vi "FSK_Sampling.vi"(8 "error in (no error)":errorcluster caption="错误输入（无错误）", 9 "pos":dbl format="%#_13g", 10 "RecvFskDemod":dbl[](array[numeric]) format="%#_13g", 11 "PathIn":path) -> (0 "error out":errorcluster caption="错误输出", 2 "RecvSymbolSampled":dbl[](array[numeric]) format="%#_13g", 3 "PathOut":path)   [LabVIEW 2015]
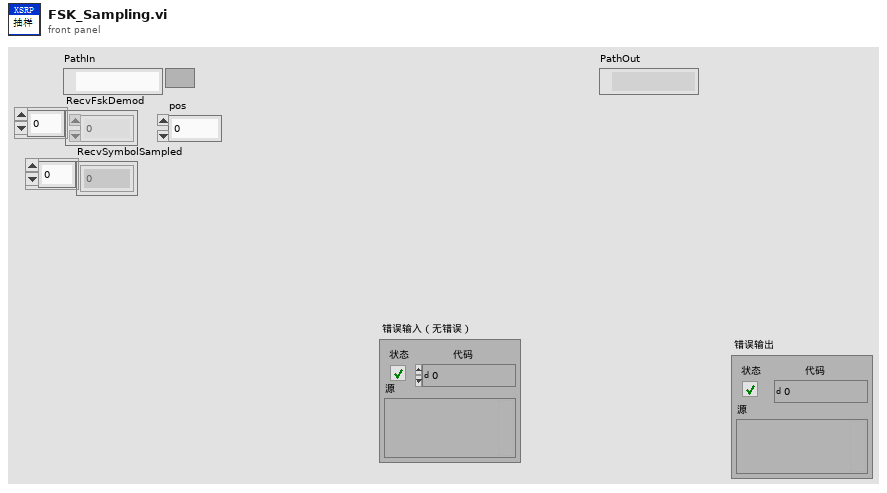
[diagram p1: front panel]
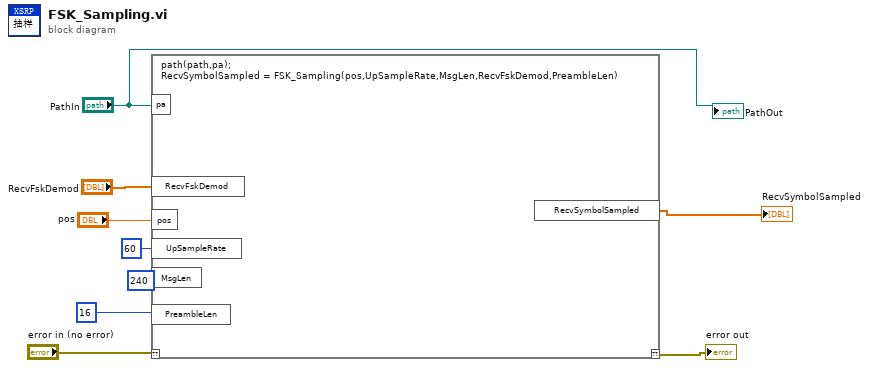
[diagram p0: block diagram]
diagram:
  n1 = script code="path(path,pa);\nRecvSymbolSampled = FSK_Sampling(pos,UpSampleRate,MsgLen,RecvFskDemod,PreambleLen)"("??"="error in (no error)", "pa"="PathIn", "RecvFskDemod"="RecvFskDemod", "pos"="pos", "UpSampleRate"=60, "MsgLen"=240, "PreambleLen"=16) -> ("??"=→"error out":errorcluster, "RecvSymbolSampled"=→"RecvSymbolSampled":dbl[])
  "PathOut" <- "PathIn"
